vi "main.vi"   [LabVIEW 2013]
uses:
  <vilib>/NXT/Remote Library/Sound/NXT_SoundVolume.ctl
  <vilib>/NXT/Dual Mode Library/Display/clearDisplay.vi
  <vilib>/NXT/Dual Mode Library/Display/drawPicture.vi
  <vilib>/NXT/Dual Mode Library/Waits/Wait_Num.vi
  <vilib>/NXT/Dual Mode Library/Sound/PlaySoundFile.vi
  <vilib>/NXT/Dual Mode Library/Advanced/NXTFlag_Assign.vi
  <vilib>/NXT/Dual Mode Library/Advanced/NXTFlag_Get_Integer.vi
  <vilib>/NXT/Dual Mode Library/Sensors/EV3_Color_Color.vi
  <vilib>/NXT/Dual Mode Library/Display/drawText_Center.vi
types:
  T1 = typedef "NXT_SoundVolume.ctl" = u8
  T2 = typedef "LVHSConnector.ctl" = refnum<class "BrickReference.lvclass">
  T3 = typedef "ColorSensorColors.ctl" = enum16{"No Color", "Black", "Blue", "Green", "Yellow", "Red", "White", "Brown"}
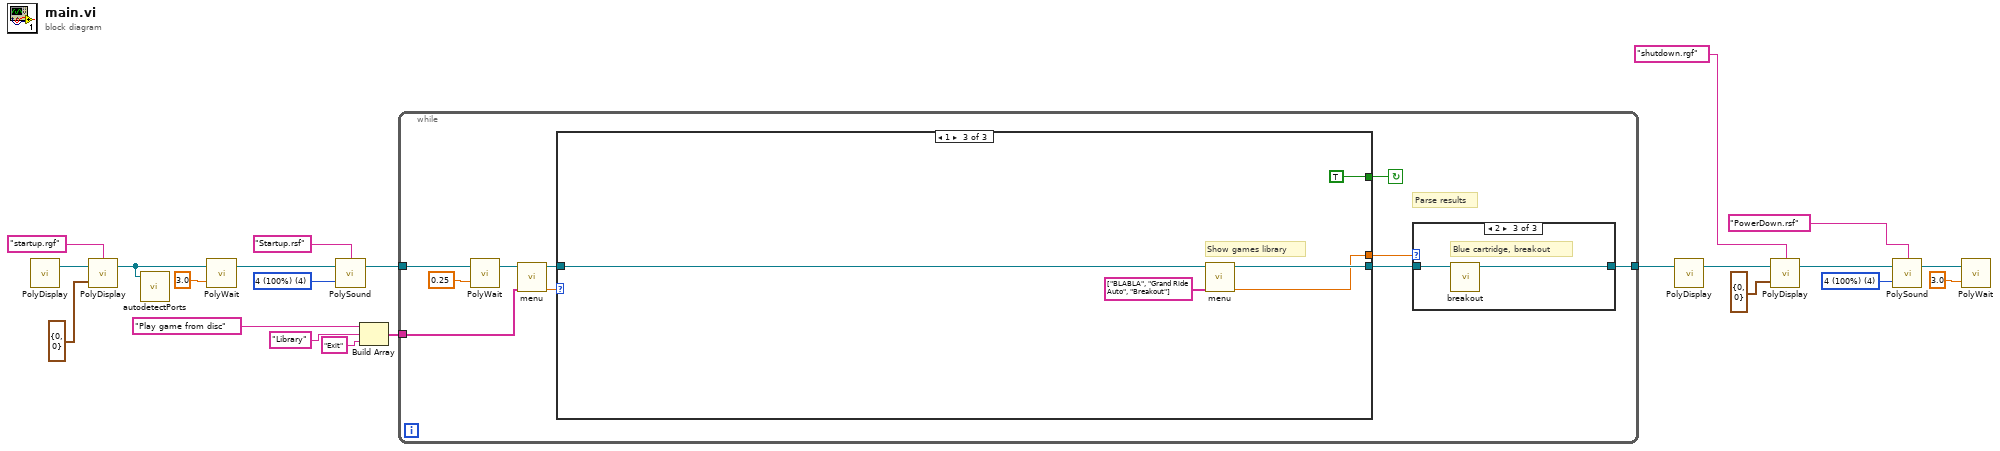
[diagram p0: block diagram]
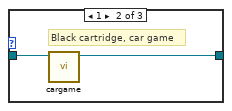
[diagram p3: hidden frame]
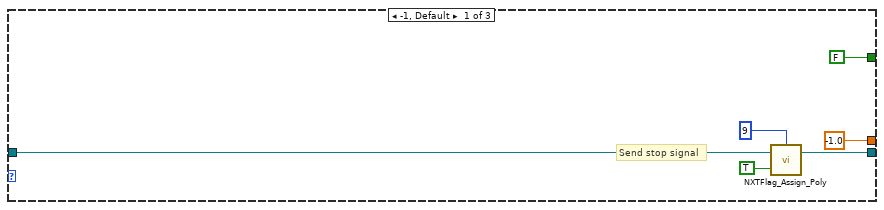
[diagram p4: hidden frame]
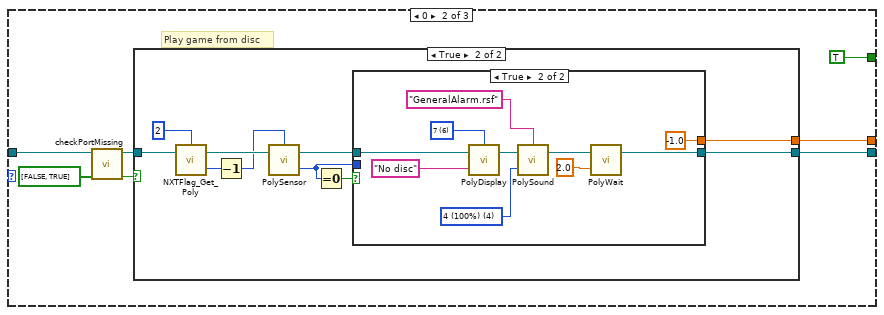
[diagram p5: hidden frame]
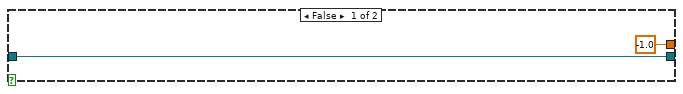
[diagram p6: hidden frame]
diagram:
  w5 = T1 4 items=["0 (Mute)", "1 (25%)", "2 (50%)", "3 (75%)", "4 (100%)"] ("Volume (4)")
  w15 = T1 4 items=["0 (Mute)", "1 (25%)", "2 (50%)", "3 (75%)", "4 (100%)"] ("Volume (4)")
  n1 = call-poly <vilib>:"PolyDisplay.vi"() -> ("NXT/EV3"=w12:T2)  [unwired: 4 in]
  n2 = call-poly <vilib>:"PolyDisplay.vi"("Origin"=cluster{"X":i16, "Y":i16} {"X"=0, "Y"=0}, "NXT/EV3"=w12, "Filename (*.ric/*.rgf)"="startup.rgf") -> ("NXT/EV3"=w17:T2)  [unwired: 1 in]
  n3 = call "autodetectPorts.vi"("NXT/EV3"=w17) -> ()  [unwired: 11 in]
  n4 = call-poly <vilib>:"PolyWait.vi"("Time (1 sec)"=sgl 3.0, "NXT/EV3"=w17) -> ("NXT/EV3"=w4:T2)  [unwired: 2 in]
  n5 = call-poly <vilib>:"PolySound.vi"("Volume (4)"=w15, "NXT/EV3"=w4, "Filename (*.rso/*.rsf)"="Startup.rsf") -> ("NXT/EV3"=w18:T2)  [unwired: 1 in]
  n6 = Build Array("Play game from disc", "Library", "Exit") -> (w19:string[])
  n7 = while {
    tunnel: w19 -> [w31]
    tunnel: w18 -> [w29]
    tunnel: [w26] -> w11
    stop <- w28 continue-if-true
    # "Parse results"
    n8 = call-poly <vilib>:"PolyWait.vi"("Time (1 sec)"=sgl 0.25, "NXT/EV3"=w29) -> ("NXT/EV3"=w24:T2)  [unwired: 2 in]
    n9 = call "menu.vi"("Elements"=w31, "NXT/EV3 2"=w24) -> ("Goto"=w30:dbl, "NXT/EV3"=w32:T2)  [unwired: 8 in]
    n10 = case shown="1" w30 {
      tunnel: w32 -> [w41 w47 w77]
      tunnel: [w40 w49 w78] -> w25
      tunnel: [FALSE TRUE TRUE] -> w28
      tunnel: [-1.0 ("Goto") w45 w75] -> w27
      frame -1, Default {
        # "Send stop signal"
        n11 = call-poly <vilib>:"NXTFlag_Assign_Poly.vi"("Flag State"=TRUE, "NXT/EV3"=w41, "NXT/EV3 Flag Number"=i8 9) -> ("NXT/EV3"=w40:T2)  [unwired: 1 in]
      }
      frame 0 {
        # "Play game from disc"
        n12 = call "checkPortMissing.vi"("Required"=bool[] [FALSE, TRUE], "NXT/EV3"=w47) -> ("Success"=w44:bool, "NXT/EV3"=w48:T2)  [unwired: 8 in]
        n13 = case shown="True" w44 {
          tunnel: [w52 w56] -> w49
          tunnel: w48 -> [w52 w62]
          tunnel: [-1.0 ("Goto") w54] -> w45
          frame False {
          }
          frame True {
            n14 = call-poly <vilib>:"NXTFlag_Get_Poly.vi"("NXT/EV3"=w62, "NXT/EV3 Flag Number"=2) -> ("Flag Value"=w60:i32, "NXT/EV3"=w59:T2)  [unwired: 1 in]
            n15 = Decrement(x=w60) -> (x-1=w58:i32)
            n16 = call-poly <vilib>:"PolySensor.vi"("NXT/EV3"=w59, "Port (Port 1)"=w58) -> ("Detected Color"=w53:T3, "NXT/EV3"=w57:T2)  [unwired: 1 in]
            n17 = Equal To 0?(x=w53) -> (x = 0?=w55:bool)
            n18 = case shown="True" w55 {
              tunnel: w57 -> [w64 w73]
              tunnel: [w64 w66] -> w56
              tunnel: [w63 -1.0 ("Goto")] -> w54
              tunnel: w53 -> [w63 _]
              frame False {
              }
              frame True {
                w68 = T1 4 items=["0 (Mute)", "1 (25%)", "2 (50%)", "3 (75%)", "4 (100%)"] ("Volume (4)")
                w71 = i16 6 items=["1", "2", "3", "4", "5", "6", "7", "8", "9", "10", "11", "12"] ("Line")
                n19 = call-poly <vilib>:"PolyDisplay.vi"("Text"="No disc", "NXT/EV3"=w73, "Line"=w71) -> ("NXT/EV3"=w72:T2)  [unwired: 1 in]
                n20 = call-poly <vilib>:"PolySound.vi"("Volume (4)"=w68, "NXT/EV3"=w72, "Filename (*.rso/*.rsf)"="GeneralAlarm.rsf") -> ("NXT/EV3"=w69:T2)  [unwired: 1 in]
                n21 = call-poly <vilib>:"PolyWait.vi"("Time (1 sec)"=sgl 2.0, "NXT/EV3"=w69) -> ("NXT/EV3"=w66:T2)  [unwired: 2 in]
              }
            }
          }
        }
      }
      frame 1 {
        # "Show games library"
        n22 = call "menu.vi"("Elements"=string[] ["BLABLA", "Grand Ride Auto", "Breakout"], "NXT/EV3 2"=w77) -> ("Goto"=w75:dbl, "NXT/EV3"=w78:T2)  [unwired: 8 in]
      }
    }
    n23 = case shown="2" w27 {
      tunnel: [w33 w35 w36] -> w26
      tunnel: w25 -> [w33 w34 w37]
      frame -1, Default {
        # "No game is to be played"
      }
      frame 1 {
        # "Black cartridge, car game"
        n24 = call "cargame.vi"("NXT/EV3"=w34) -> ("NXT/EV3 2"=w35:T2)  [unwired: 10 in]
      }
      frame 2 {
        # "Blue cartridge, breakout"
        n25 = call "breakout.vi"("NXT/EV3"=w37) -> ("NXT/EV3 2"=w36:T2)  [unwired: 10 in]
      }
    }
  }
  n26 = call-poly <vilib>:"PolyDisplay.vi"("NXT/EV3"=w11) -> ("NXT/EV3"=w10:T2)  [unwired: 3 in]
  n27 = call-poly <vilib>:"PolyDisplay.vi"("Origin"=cluster{"X":i16, "Y":i16} {"X"=0, "Y"=0}, "NXT/EV3"=w10, "Filename (*.ric/*.rgf)"="shutdown.rgf") -> ("NXT/EV3"=w7:T2)  [unwired: 1 in]
  n28 = call-poly <vilib>:"PolySound.vi"("Volume (4)"=w5, "NXT/EV3"=w7, "Filename (*.rso/*.rsf)"="PowerDown.rsf") -> ("NXT/EV3"=w2:T2)  [unwired: 1 in]
  n29 = call-poly <vilib>:"PolyWait.vi"("Time (1 sec)"=sgl 3.0, "NXT/EV3"=w2) -> ()  [unwired: 2 in, 1 out]
